vi "Write.vi"(8 "error in (no error)":errorcluster, 10 "Data":dbl[](array[numeric]), 11 "Test Double Data in":refnum<class "Test Double Data.lvclass">) -> (0 "error out":errorcluster, 3 "Test Double Data out":refnum<class "Test Double Data.lvclass">)   [LabVIEW 2020, in "Test.lvlib" / "Test Double Data.lvclass"]
uses:
  Test Double Data.lvclass
  Test Double Data.lvclass/Test Double Data.ctl
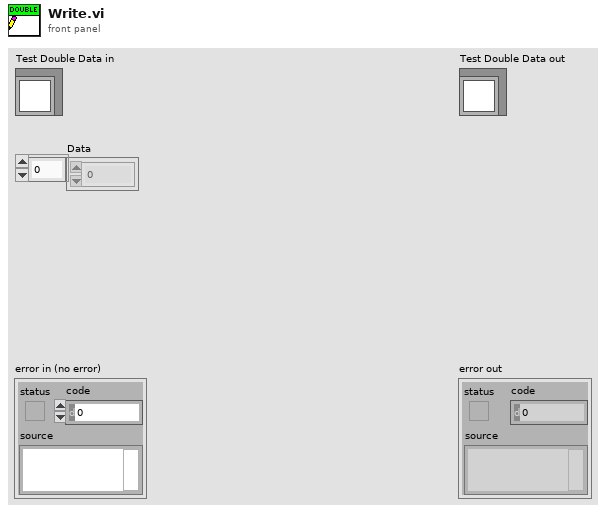
[diagram p1: front panel]
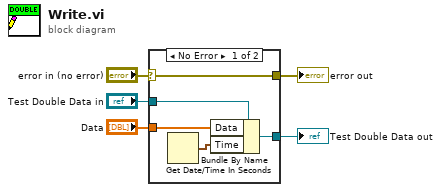
[diagram p0: block diagram]
diagram:
  n1 = case shown="No Error" "error in (no error)" {
    selector: "error in (no error)" -> [w10 w11]
    tunnel: [w10 w11] -> w4
    tunnel: [w8 w12] -> w2
    tunnel: "Test Double Data in" -> [w9 w12]
    tunnel: "Data" -> [w7 _]
    frame No Error {
      n2 = Get Date/Time In Seconds() -> (seconds since 1Jan1904=w6:timestamp)
      n3 = Bundle By Name(cluster=w9, "Data"=w7, "Time"=w6) -> (w8:refnum<class "Test Double Data.lvclass">)
    }
    frame Error {
    }
  }
  "error out" <- w4
  "Test Double Data out" <- w2
